vi "T1 Parametric Testing.vi"(5 "error in":errorcluster, 6 "Operator":string, 7 "table name":string="Test_Results", 8 "connection reference":T1) -> (0 "error out":errorcluster, 3 "connection reference out":T1)   [LabVIEW 2013]
doc: "The T1 Parametric testing application performs parametric testing of T1 signals. The T1 signal is a 1.544 Mb/s pulsed digital signal formed by multiplexing 24 voice channels. Each channel is sampled at 8000 samples/sec. Each sample is then converted to 8 bits using Pulse Coded Multiplexing. The 24 channels are then time-division multiplexed. Each frame, which corresponds to one sampling period, contains 192 bits ( 8 times 24) plus one bit for frame synchronization. Since frames occur at 8000 times per second, the bit rate is 1.544 Mb/s\n\nThis application performs the following parametric tests on T1 signals:\n\n1. Mask Test: Compares T1 signals with standard masks. The type of masks that are supported are ITU G.703 mask, EIA/TIA 547 and ANSI T1.102. The graph shows the mask in grey, the actual signal in green and failures as red squares. A boolean indicates whether the signal passed or failed the mask test and the indicator Number of Hits shows the number of times the signal did not pass the mask test.\n\n2. Measure T1 signal amplitude : Measures the amplitude of the T1 signal. The peak amplitude is displayed in the indicator Measured Amplitude.\n\n3. Measure T1 signal frequency : Measures the frequency of the T1 signal. The signal frequency in MHz is displayed in the indicator Measured Frequency."
uses:
  Connection.llb/Conn ObjectReference.ctl
  Auxilliary.llb/DB Tools Column Info.ctl
  Auxilliary.llb/DB Tools DataTypes.ctl
  NI_Database_API_64.lvlib
panel:
  out "Passed?":bool
  in  "Log to Database":bool
  in  "Start Testing":bool
  out "Standard":string
  out "Date/Time":string
  out "UUT Serial #":string
  out "Failures":i32(slide) scale=0.0..10.0
  out "Tests":i32(slide) scale=0.0..10.0
  in  "quit":bool
  out "Amplitude (Vrms)":dbl(knob) scale=0.0..3.0 scale format="%.1f"
  in  "Polarity":bool=TRUE
  out "Frequency (MHz)":dbl format="%.4f"
  out "Time Domain Signal":waveform(dbl)(graph)
  out "Amplitude Spectrum":T2(graph)
  out "Signal Mask Test":waveform(dbl)[](graph)
  # "Telecommunications Parametric Testing"
  # "+"
  # "-"
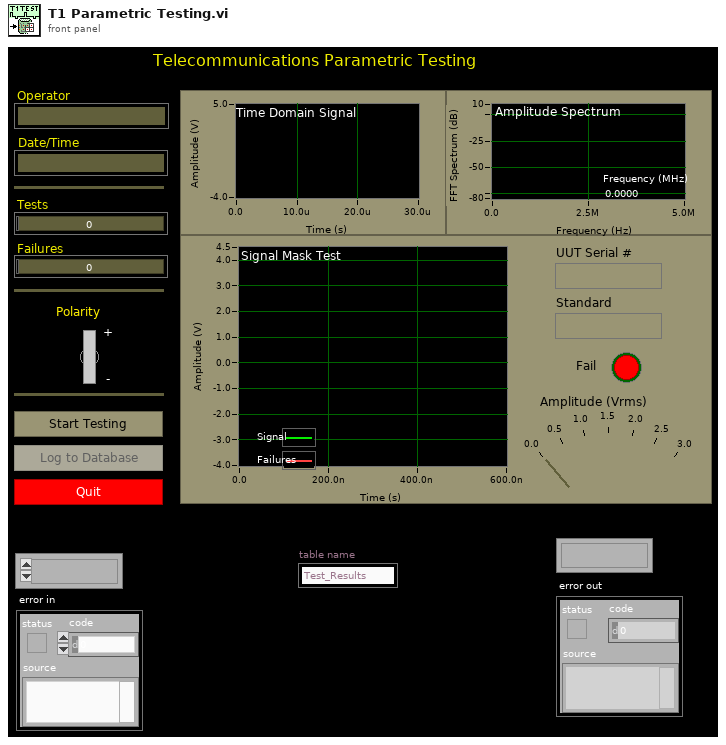
[diagram p1: front panel]
types:
  T1 = typedef "NI_Database_API_64.lvlib/Conn ObjectReference.ctl" = refnum<k1>
  T2 = cluster{"f0":dbl, "df":dbl, "dB Spectrum (Hann)":dbl[]}
  T3 = enum16{"Init", "Testing", "Logging", "Idle", "Quit"}
  T4 = typedef "NI_Database_API_64.lvlib/DB Tools Column Info.ctl" = cluster{"column name":string, "data type":T5, "size":i32, "allow null?":bool}
  T5 = typedef "NI_Database_API_64.lvlib/DB Tools DataTypes.ctl" = enum16{"String", "Long (I32)", "Single (SGL)", "Double (DBL)", "Date/Time", "Binary"}
  T6 = cluster{"Time Domain Signal":waveform(dbl), "Signal Mask Test":waveform(dbl)[], "Amplitude (Vrms)":dbl, "Frequency (MHz)":dbl, "Date/Time":string, "Passed?":bool}
  T7 = cluster{"Operator":string, "UUT Serial #":string, "UUT Serial #":string, "UUT Serial #":string, dbl, "UUT Serial #":string, "UUT Serial #":string}
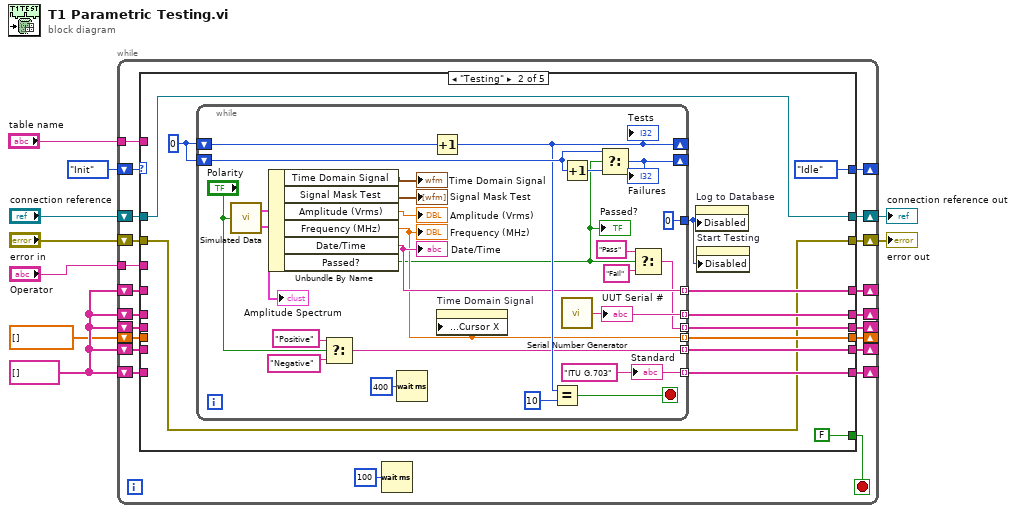
[diagram p0: block diagram]
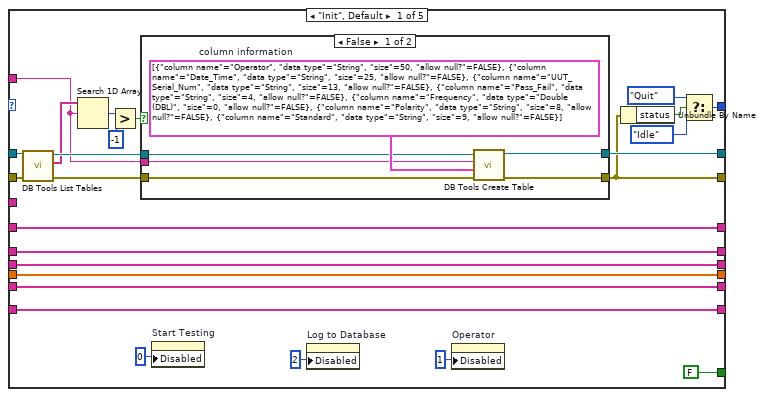
[diagram p2: hidden frame]
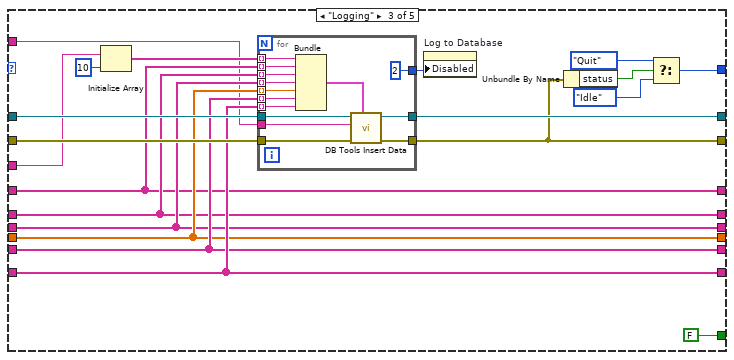
[diagram p4: hidden frame]
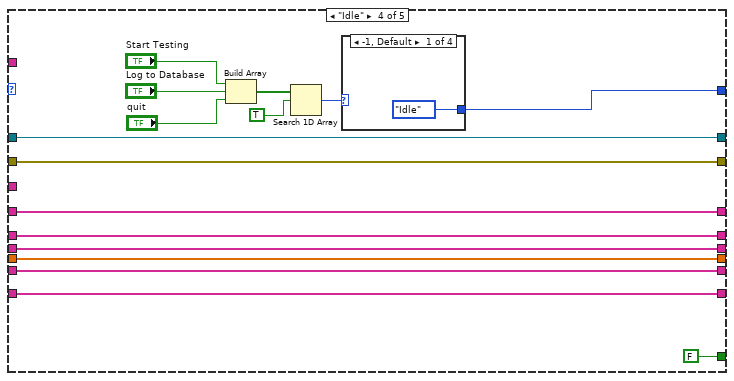
[diagram p5: hidden frame]
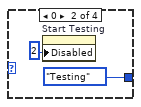
[diagram p6: hidden frame]
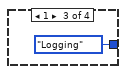
[diagram p7: hidden frame]
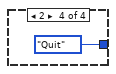
[diagram p8: hidden frame]
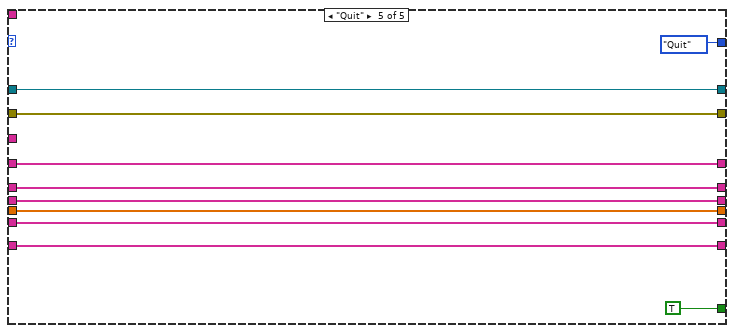
[diagram p9: hidden frame]
diagram:
  w9 = string[] []
  n1 = while {
    tunnel: "table name" -> [w10]
    tunnel: "Operator" -> [w11]
    shift-left: T3."Init" ("initial state") -> [w14]
    shift-right: [w13] -> _
    shift-left: "error in" -> [w16]
    shift-right: [w17] -> w4
    shift-left: "connection reference" -> [w15]
    shift-right: [w18] -> w3
    shift-left: w9 -> [w26]
    shift-right: [w19] -> _
    shift-left: w9 -> [w27]
    shift-right: [w20] -> _
    shift-left: dbl[] [] -> [w28]
    shift-right: [w21] -> _
    shift-left: w9 -> [w29]
    shift-right: [w22] -> _
    shift-left: w9 -> [w30]
    shift-right: [w23] -> _
    shift-left: w9 -> [w25]
    shift-right: [w24] -> _
    stop <- w12 stop-if-true
    n2 = case shown="\"Testing\"" w14 {
      tunnel: [w56 w73 w114 w143 w161] -> w23
      tunnel: [w55 w76 w115 w142 w162] -> w22
      tunnel: [w54 w71 w116 w141 w163] -> w21
      tunnel: [w53 w75 w117 w140 w164] -> w20
      tunnel: [w52 w74 w118 w139 w165] -> w19
      tunnel: w30 -> [w56 _ w114 w143 w161]
      tunnel: w29 -> [w55 _ w115 w142 w162]
      tunnel: w28 -> [w54 _ w116 w141 w163]
      tunnel: w27 -> [w53 _ w117 w140 w164]
      tunnel: w26 -> [w52 _ w118 w139 w165]
      tunnel: w25 -> [w51 _ w113 w144 w160]
      tunnel: [w51 w72 w113 w144 w160] -> w24
      tunnel: [w50 w69 w122 w146 w159] -> w18
      tunnel: [w49 w70 w105 w145 w158] -> w17
      tunnel: w16 -> [w39 w70 w119 w145 w158]
      tunnel: w15 -> [w40 w69 w121 w146 w159]
      tunnel: w11 -> [_ _ w110 _ _]
      tunnel: [w46 T3."Idle" ("state") w120 w147 T3."Quit" ("state")] -> w13
      tunnel: [FALSE FALSE FALSE FALSE TRUE] -> w12
      tunnel: w10 -> [w33 _ w103 _ _]
      frame "Init", Default {
        n3 = call "DB Tools List Tables.vi"("error in (no error)"=w39, "connection reference"=w40) -> ("error out"=w35:errorcluster, "tables"=w34:string[], "connection reference out"=w36:T1)  [unwired: 3 in]
        n4 = Search 1D Array(1D array=w34, element=w33) -> (index of element=w37:i32)  [unwired: 1 in]
        n5 = Greater?(x=w37, y=-1) -> (0:w32:bool)
        n6 = case shown="False" w32 {
          tunnel: [w62 w64] -> w50
          tunnel: [w60 w63] -> w49
          tunnel: w33 -> [w59 _]
          tunnel: w36 -> [w58 w64]
          tunnel: w35 -> [w57 w63]
          frame False {
            w61 = T4[] [{"column name"="Operator", "data type"=enum."String", "size"=50, "allow null?"=FALSE}, {"column name"="Date_Time", "data type"=enum."String", "size"=25, "allow null?"=FALSE}, {"column name"="UUT_Serial_Num", "data type"=enum."String", "size"=13, "allow null?"=FALSE}, {"column name"="Pass_Fail", "data type"=enum."String", "size"=4, "allow null?"=FALSE}, {"column name"="Frequency", "data type"=enum."Double (DBL)", "size"=0, "allow null?"=FALSE}, {"column name"="Polarity", "data type"=enum."String", "size"=8, "allow null?"=FALSE}, {"column name"="Standard", "data type"=enum."String", "size"=9, "allow null?"=FALSE}]  # column information
            n7 = call "DB Tools Create Table.vi"("error in (no error)"=w57, "column information"=w61, "table"=w59, "connection reference"=w58) -> ("error out"=w60:errorcluster, "connection reference out"=w62:T1)  [unwired: 4 in]
          }
          frame True {
          }
        }
        n8 = property on="Start Testing" class="Bool"("Disabled"=u8 0) -> ()  [unwired: 2 in, 2 out]
        n9 = property on="Log to Database" class="Bool"("Disabled"=u8 2) -> ()  [unwired: 2 in, 2 out]
        n10 = property on="Operator" class="Str"("Disabled"=u8 1) -> ()  [unwired: 2 in, 2 out]
        n11 = Unbundle By Name(w49) -> ("status"=w48:bool)
        n12 = Select(t=T3."Quit" ("state"), s=w48, f=T3."Idle" ("state")) -> (s? t:f=w46:T3)
      }
      frame "Testing" {
        w66 = 0
        n13 = while {
          tunnel: [u8 0 ("Disabled")] -> w65
          tunnel: [w87] -> w71 mode=indexing
          tunnel: [w88] -> w72 mode=indexing
          tunnel: [w99] -> w74 mode=indexing
          tunnel: [w86] -> w75 mode=indexing
          tunnel: [w81] -> w76 mode=indexing
          tunnel: [w100] -> w73 mode=indexing
          shift-left: w66 -> [w95]
          shift-right: [w94] -> _
          shift-left: w66 -> [w96]
          shift-right: [w77] -> _
          stop <- w102 stop-if-true
          w99 = "ITU G.703" ("Standard")
          n14 = call "Simulated Data.vi"("Polarity"="Polarity") -> ("Cluster"=w92:T6, "Amplitude Spectrum"=→"Amplitude Spectrum":T2)
          n15 = Unbundle By Name(w92) -> ("Time Domain Signal"=→"Time Domain Signal":waveform(dbl), "Signal Mask Test"=→"Signal Mask Test":waveform(dbl)[], "Amplitude (Vrms)"=→"Amplitude (Vrms)":dbl, "Frequency (MHz)"=w87:dbl, "Date/Time"=w88:string, "Passed?"=w82:bool)
          "Frequency (MHz)" <- w87
          "Passed?" <- w82
          "Date/Time" <- w88
          n16 = Select(t="Positive", s="Polarity", f="Negative") -> (s? t:f=w86:string)
          n17 = Wait (ms)(milliseconds to wait=u32 400) -> ()  [unwired: 1 out]
          n18 = Increment(x=w95) -> (x+1=w94:i32)
          "Tests" <- w94
          n19 = property on="Time Domain Signal" class="WFGraph (strict)"("Cursor.Cursor Position:Cursor X"=w87) -> ()  [unwired: 2 in, 2 out]
          n20 = Equal?(x=w94, y=10 ("x")) -> (x = y?=w102:bool)
          n21 = Increment(x=w96) -> (x+1=w97:i32)
          n22 = call "Serial Number Generator.vi"() -> ("UUT Serial #"=w100:string)
          "UUT Serial #" <- w100
          n23 = Select(t=w96, s=w82, f=w97) -> (s? t:f=w77:i32)
          "Failures" <- w77
          n24 = Select(t="Pass", s=w82, f="Fail") -> (s? t:f=w81:string)
          "Standard" <- w99
        }
        n25 = property on="Log to Database" class="Bool"("Disabled"=w65) -> ()  [unwired: 2 in, 2 out]
        n26 = property on="Start Testing" class="Bool"("Disabled"=w65) -> ()  [unwired: 2 in, 2 out]
      }
      frame "Logging" {
        n27 = Initialize Array(w110, 10 ("Dimension Size")) -> (w109:string[])
        n28 = for {
          tunnel: [w135] -> w122
          tunnel: [w134] -> w105
          tunnel: w109 -> [w133] mode=indexing
          tunnel: w113 -> [w132] mode=indexing
          tunnel: w114 -> [w131] mode=indexing
          tunnel: w115 -> [w130] mode=indexing
          tunnel: w116 -> [w129] mode=indexing
          tunnel: w117 -> [w128] mode=indexing
          tunnel: w118 -> [w127] mode=indexing
          tunnel: w121 -> [w126]
          tunnel: w119 -> [w125]
          tunnel: [u8 2 ("Disabled")] -> w112
          tunnel: w103 -> [w123]
          n29 = Bundle("Operator"=w133, "UUT Serial #"=w132, "UUT Serial #"=w131, "UUT Serial #"=w130, w129, "UUT Serial #"=w128, "UUT Serial #"=w127) -> (w136:T7)  [unwired: 1 in]
          n30 = call "DB Tools Insert Data.vi"("data"=w136, "error in (no error)"=w125, "table"=w123, "connection reference"=w126) -> ("error out"=w134:errorcluster, "connection reference out"=w135:T1)  [unwired: 6 in]
        }
        n31 = property on="Log to Database" class="Bool"("Disabled"=w112) -> ()  [unwired: 2 in, 2 out]
        n32 = Unbundle By Name(w105) -> ("status"=w107:bool)
        n33 = Select(t=T3."Quit" ("state"), s=w107, f=T3."Idle" ("state")) -> (s? t:f=w120:T3)
      }
      frame "Idle" {
        n34 = Build Array("Start Testing", "Log to Database", "quit") -> (w150:bool[])
        n35 = Search 1D Array(1D array=w150, element=TRUE) -> (index of element=w148:i32)  [unwired: 1 in]
        n36 = case shown="-1, Default" w148 {
          tunnel: [T3."Idle" ("state") T3."Testing" ("state") T3."Logging" ("state") T3."Quit" ("state")] -> w147
          frame -1, Default {
          }
          frame 0 {
            n37 = property on="Start Testing" class="Bool"("Disabled"=u8 2) -> ()  [unwired: 2 in, 2 out]
          }
          frame 1 {
          }
          frame 2 {
          }
        }
      }
      frame "Quit" {
      }
    }
    n38 = Wait (ms)(milliseconds to wait=u32 100) -> ()  [unwired: 1 out]
  }
  "connection reference out" <- w3
  "error out" <- w4
